vi "Launch Actors.vi"(8 "error in (no error)":errorcluster, 10 "Actor":enum16{"Mixer", "Screw", "Solenoid", "All"}(ring), 11 "Feeder Actor.lvlib:Feeder.lvclass":refnum<class "Feeder.lvclass">) -> (0 "error out":errorcluster, 3 "Feeder Actor.lvlib:Feeder.lvclass 2":refnum<class "Feeder.lvclass">)   [LabVIEW 2018, in "Feeder Actor.lvlib" / "Feeder.lvclass"]
uses:
  Feeder.lvclass
  Feeder.lvclass/Feeder.ctl
  Solenoid/Solenoid.lvclass
  Counter/Counter.lvclass
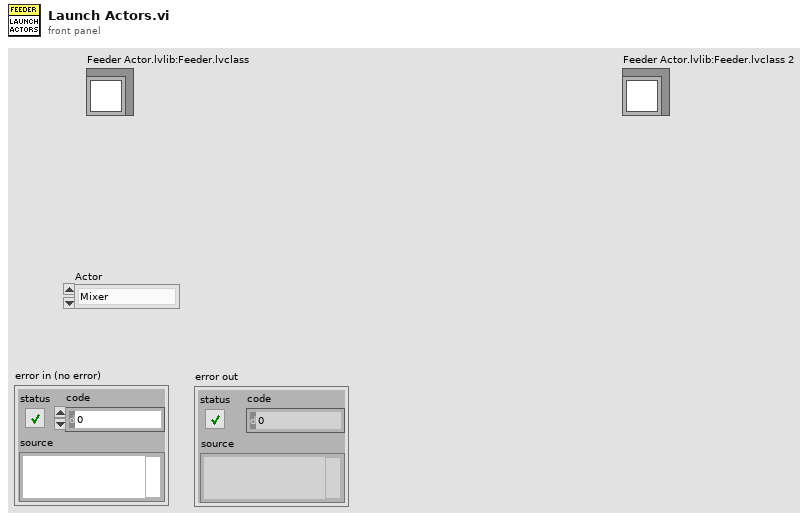
[diagram p1: front panel]
types:
  T1 = cluster{"Mixer":refnum<vi>, "Screw":refnum<vi>, "Solenoid":refnum<vi>}
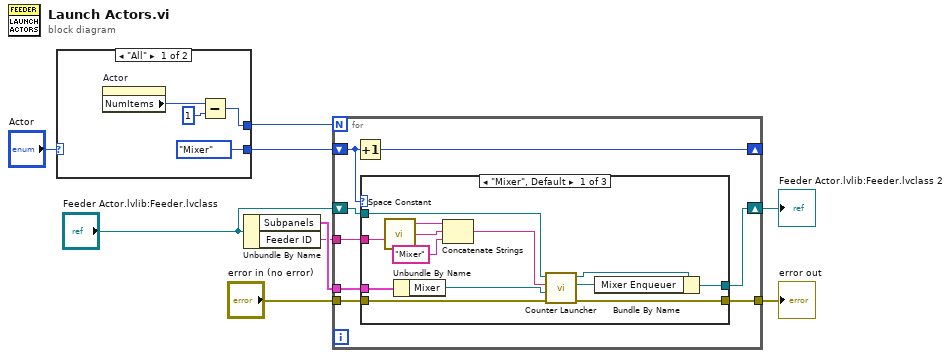
[diagram p0: block diagram]
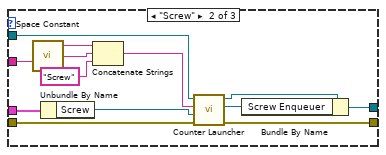
[diagram p2: hidden frame]
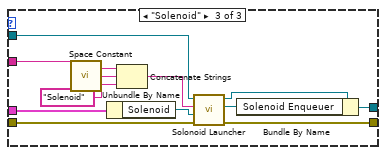
[diagram p3: hidden frame]
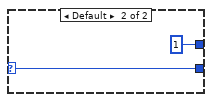
[diagram p4: hidden frame]
diagram:
  n1 = case shown="\"All\"" "Actor" {
    selector: "Actor" -> [_ w14]
    tunnel: [w13 1] -> w8
    tunnel: [enum16{"Mixer", "Screw", "Solenoid", "All"}."Mixer" ("Actor 2") w14] -> w9
    frame "All" {
      n2 = property on="Actor" class="Enum (strict)"() -> ("NumItems"=w11:u32)  [unwired: 2 in, 2 out]
      n3 = Subtract(x=w11, y=u32 1) -> (x-y=w13:u32)
    }
    frame Default {
    }
  }
  n4 = Unbundle By Name("Feeder Actor.lvlib:Feeder.lvclass") -> ("Subpanels"=w7:T1, "Feeder ID"=w1:string)
  n5 = for {
    N: w8 -> [_]
    shift-right: [w23] -> _
    shift-left: w9 -> [w22]
    shift-right: [w17] -> w4
    shift-left: "Feeder Actor.lvlib:Feeder.lvclass" -> [w21]
    tunnel: w7 -> [w20]
    tunnel: "error in (no error)" -> [w19]
    tunnel: [w18] -> w5
    tunnel: w1 -> [w16]
    n6 = Increment(x=w22) -> (x+1=w23:enum16{"Mixer", "Screw", "Solenoid", "All"})
    n7 = case shown="\"Mixer\", Default" w22 {
      tunnel: w21 -> [w32 w44 w53]
      tunnel: w20 -> [w35 w47 w59]
      tunnel: [w34 w46 w51] -> w17
      tunnel: w19 -> [w30 w42 w49]
      tunnel: [w29 w41 w48] -> w18
      tunnel: w16 -> [w24 w37 w57]
      frame "Mixer", Default {
        n8 = call <vilib>:"Space Constant.vi"() -> ("String"=w26:string)
        n9 = Unbundle By Name(w35) -> ("Mixer"=w31:refnum<vi>)
        n10 = Concatenate Strings(w24, w26, "Mixer") -> (w25:string)
        n11 = call "Counter Launcher.vi"("error in (no error)"=w30, "Sub Panel"=w31, "Counter ID"=w25, "Feeder Actor In"=w32) -> ("error out"=w29:errorcluster, "Nested Actor's Enqueuer"=w33:refnum<class "Message Enqueuer.lvclass">, "Feeder Actor Out"=w28:refnum<class "Feeder.lvclass">)  [unwired: 5 in]
        n12 = Bundle By Name(cluster=w28, "Mixer Enqueuer"=w33) -> (w34:refnum<class "Feeder.lvclass">)
      }
      frame "Screw" {
        n13 = call <vilib>:"Space Constant.vi"() -> ("String"=w36:string)
        n14 = Unbundle By Name(w47) -> ("Screw"=w43:refnum<vi>)
        n15 = Concatenate Strings(w37, w36, "Screw") -> (w38:string)
        n16 = call "Counter Launcher.vi"("error in (no error)"=w42, "Sub Panel"=w43, "Counter ID"=w38, "Feeder Actor In"=w44) -> ("error out"=w41:errorcluster, "Nested Actor's Enqueuer"=w45:refnum<class "Message Enqueuer.lvclass">, "Feeder Actor Out"=w40:refnum<class "Feeder.lvclass">)  [unwired: 5 in]
        n17 = Bundle By Name(cluster=w40, "Screw Enqueuer"=w45) -> (w46:refnum<class "Feeder.lvclass">)
      }
      frame "Solenoid" {
        n18 = call <vilib>:"Space Constant.vi"() -> ("String"=w56:string)
        n19 = Unbundle By Name(w59) -> ("Solenoid"=w54:refnum<vi>)
        n20 = Concatenate Strings(w57, w56, "Solenoid") -> (w55:string)
        n21 = call "Solonoid Launcher.vi"("error in (no error)"=w49, "Sub Panel"=w54, "Solenoid ID"=w55, "Feeder Actor In"=w53) -> ("error out"=w48:errorcluster, "Nested Actor's Enqueuer"=w50:refnum<class "Message Enqueuer.lvclass">, "Feeder Actor Out"=w52:refnum<class "Feeder.lvclass">)  [unwired: 5 in]
        n22 = Bundle By Name(cluster=w52, "Solenoid Enqueuer"=w50) -> (w51:refnum<class "Feeder.lvclass">)
      }
    }
  }
  "error out" <- w5
  "Feeder Actor.lvlib:Feeder.lvclass 2" <- w4
